vi "数据表-写入或修改记录.vi"(6 "元素名[]-探测器信息":string[](array[string]), 7 "元素名[]-累积记录":string[](array[string]), 8 "error in (no error)":errorcluster, 9 "表名-设备表":string, 10 "写改记录数据输入":T1, 11 "数据库引用":T7) -> (0 "error out":errorcluster, 1 "输出簇":T1, 2 "累积剂量增量":dbl, 3 "connection reference out":T7)   [LabVIEW 2017]
uses:
  <vilib>/addons/database/Connection.llb/Conn ObjectReference.ctl
  <vilib>/addons/database/NI_Database_API.lvlib
panel:
  out "Result 2":string caption="设备表sql-update"
  out "Result":string caption="数据表sql-update"
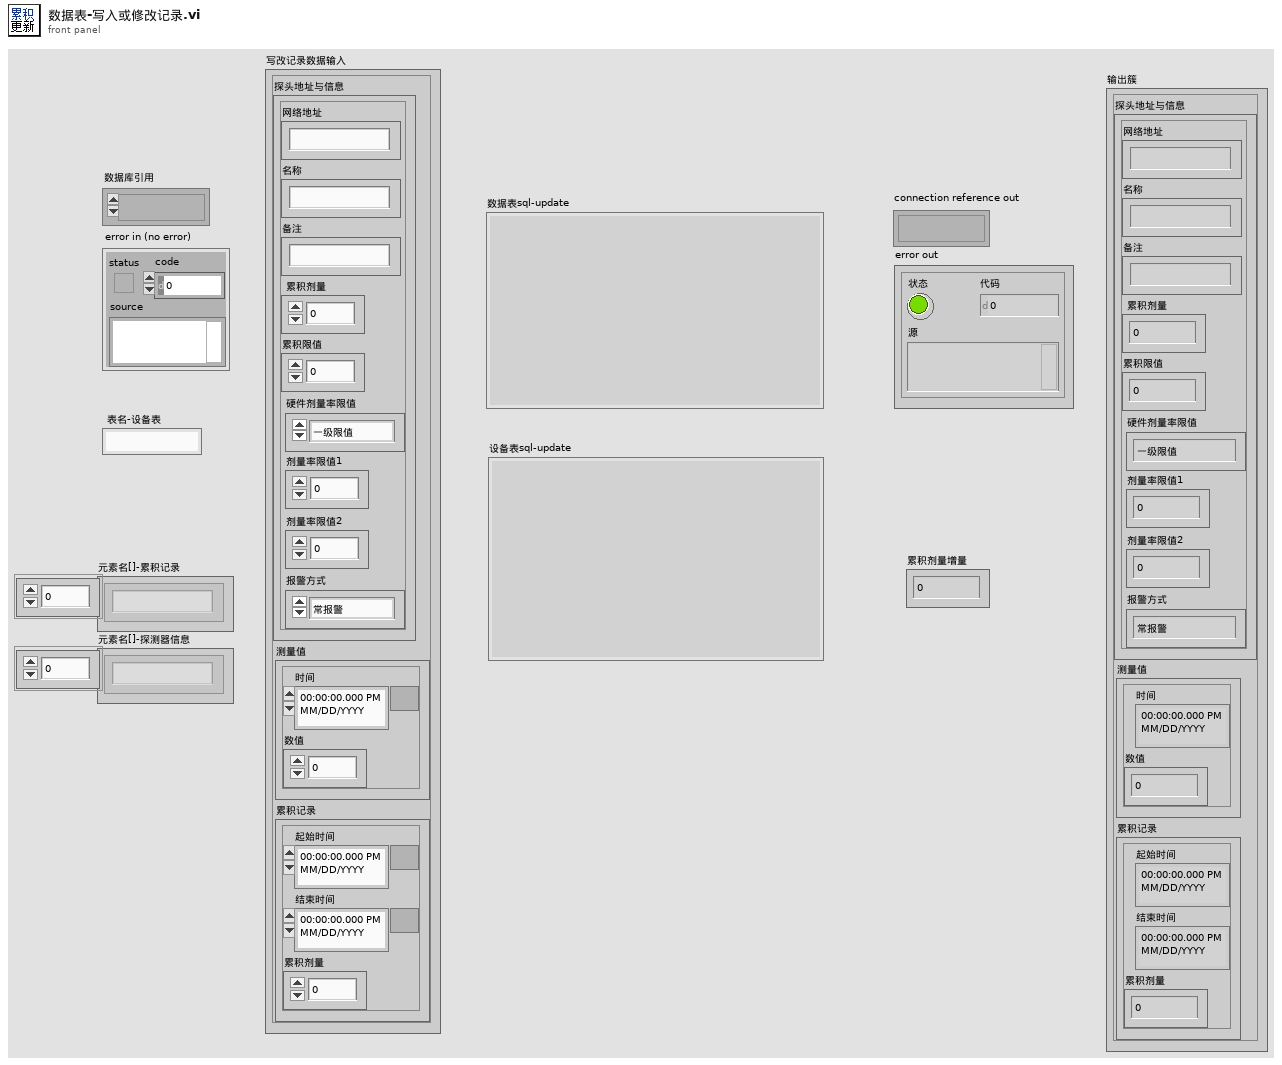
[diagram p1: front panel]
types:
  T1 = typedef "写改累积记录输入.ctl" = cluster{"探头地址与信息":T2, "测量值":T5, "累积记录":T6}
  T2 = typedef "探测器信息.ctl" = cluster{"网络地址":string, "名称":string, "备注":string, "累积剂量":dbl, "累积限值":dbl, "硬件剂量率限值":T3, "剂量率限值1":dbl, "剂量率限值2":dbl, "报警方式":T4}
  T3 = typedef "探头剂量率限值选择.ctl" = enum16{"一级限值", "二级限值"}
  T4 = typedef "报警方式选择.ctl" = enum16{"常报警", "自动静音", "手动静音"}
  T5 = typedef "测量值.ctl" = cluster{"时间":timestamp, "数值":dbl}
  T6 = typedef "单条累积记录.ctl" = cluster{"起始时间":timestamp, "结束时间":timestamp, "累积剂量":dbl}
  T7 = typedef "NI_Database_API.lvlib/Conn ObjectReference.ctl" = refnum<k1>
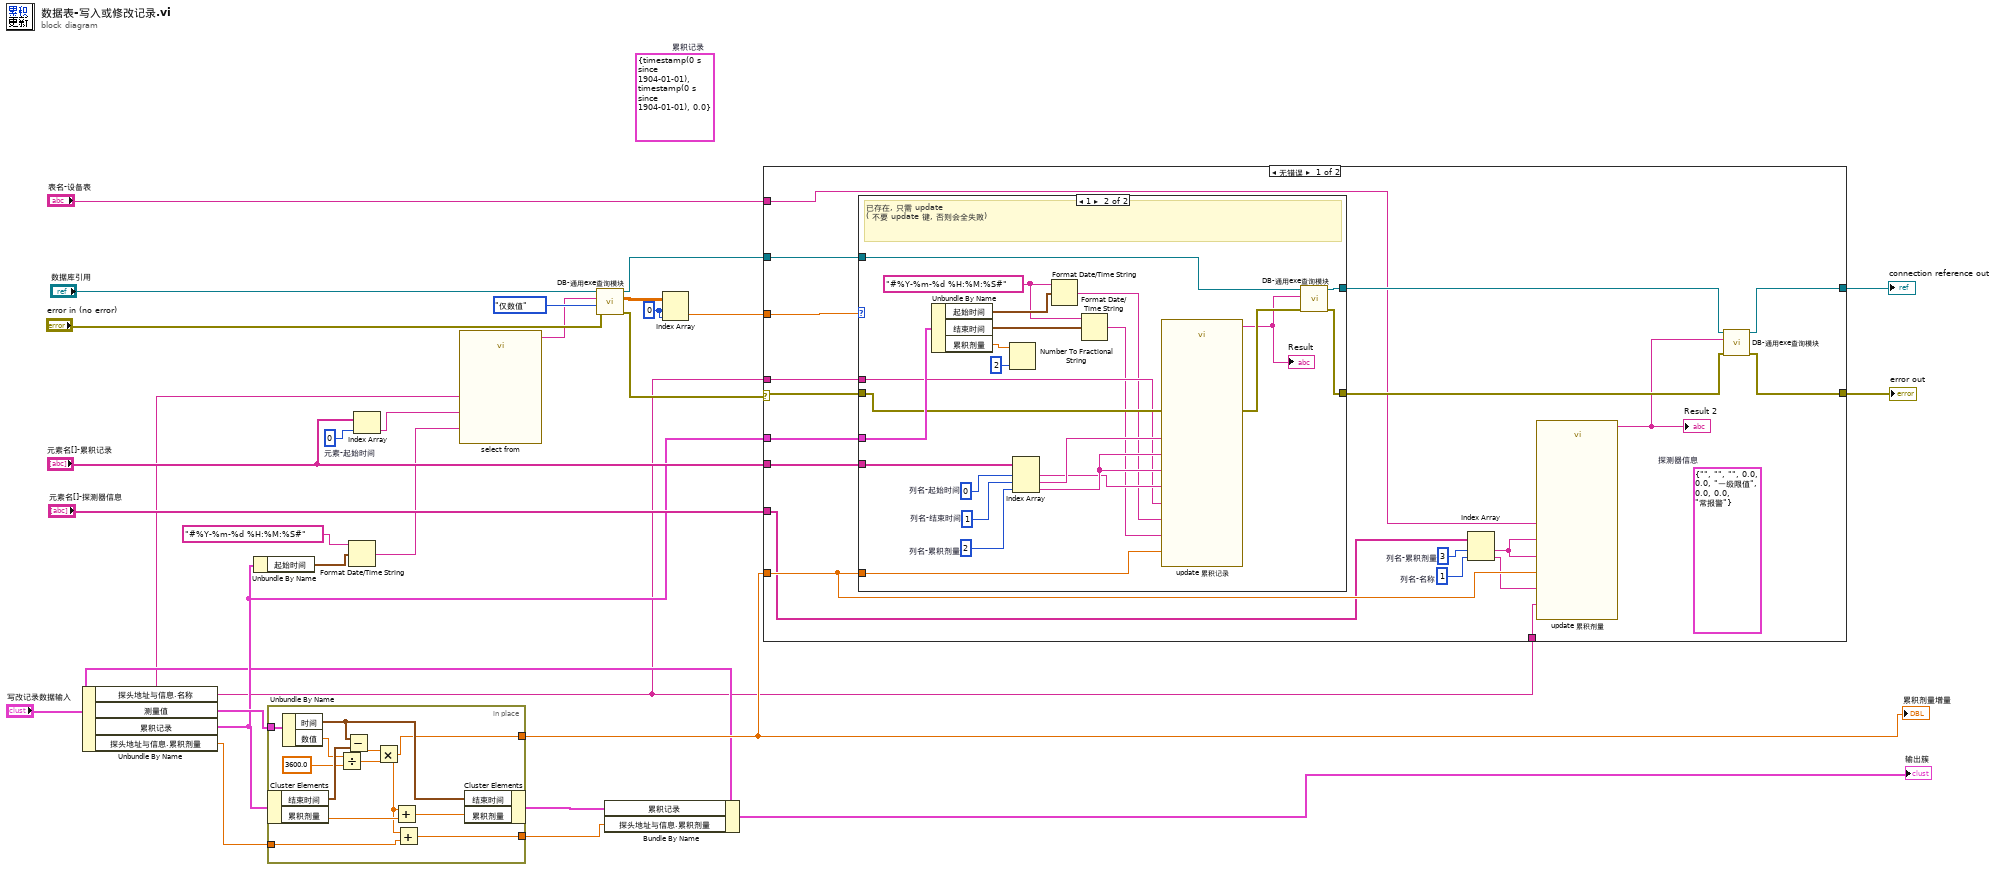
[diagram p0: block diagram]
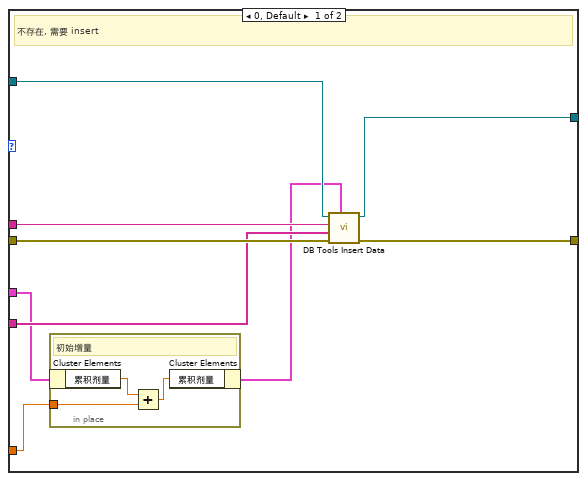
[diagram p2: hidden frame]
diagram:
  (unwired) T6 {"起始时间"=timestamp(0 s since 1904-01-01), "结束时间"=timestamp(0 s since 1904-01-01), "累积剂量"=0.0}  # 累积记录
  w22 = 0 ("索引 (行)")
  w27 = 0  # 元素-起始时间
  n1 = Unbundle By Name("写改记录数据输入") -> ("探头地址与信息.名称"=w1:string, "测量值"=w14:T5, "累积记录"=w11:T6, "探头地址与信息.累积剂量"=w3:dbl)
  n2 = Unbundle By Name(w11) -> ("起始时间"=w26:timestamp)
  n3 = in-place {
    in-place-border: w14 -> [w40]
    in-place-border: [w30] -> w7
    in-place-border: w3 -> [w31]
    in-place-border: [w29] -> w2
    n4 = in-place-cluster #1(w11) -> ("结束时间"=w38:timestamp, "累积剂量"=w39:dbl)
    n5 = Unbundle By Name(w40) -> ("时间"=w34:timestamp, "数值"=w36:dbl)
    n6 = Divide(x=w36, y=3600.0) -> (x/y=w33:dbl)
    n7 = Subtract(x=w34, y=w38) -> (x-y=w37:dbl)
    n8 = Multiply(x=w37, y=w33) -> (x*y=w30:dbl)
    n9 = Add(x=w30, y=w39) -> (x+y=w35:dbl)
    n10 = Add(x=w30, y=w31) -> (x+y=w29:dbl)
    n11 = in-place-cluster #1("结束时间"=w34, "累积剂量"=w35) -> (w5:T6)
  }
  "累积剂量增量" <- w7
  n12 = Format Date/Time String(time format string (%c)="#%Y-%m-%d %H:%M:%S#" ("时间格式字符串(%c)"), seconds (now)=w26) -> (date/time string=w9:string)  [unwired: 1 in]
  n13 = Index Array(array="元素名[]-累积记录", index=w27) -> (element=w10:string)
  n14 = call "select from"("表名"=w1, "列名-起始时间"=w9, "时间字符串"=w10) -> ("Result"=w8:string)  [unwired: 11 in, 1 out]
  n15 = call "DB-通用exe查询模块.vi"("error in (no error)"="error in (no error)", "解析模式"=enum16{"仅数值", "仅字符串", "数值与字符串"}."仅数值", "SQL query"=w8, "数据库连接引用"="数据库引用") -> ("error out"=w19:errorcluster, "数值数据"=w23:dbl[][], "数据库连接引用out"=w18:T7)  [unwired: 3 in, 2 out]
  n16 = Bundle By Name(cluster="写改记录数据输入", "累积记录"=w5, "探头地址与信息.累积剂量"=w2) -> (→"输出簇":T1)
  n17 = Index Array(array=w23, index (row)=w22, index (col)=w22) -> (element=w21:dbl)
  n18 = case shown="无错误" w19 {
    selector: w19 -> [w57 w95]
    tunnel: w21 -> [w59 _]
    tunnel: w18 -> [w58 w94]
    tunnel: [w52 w94] -> w15
    tunnel: [w50 w95] -> w17
    tunnel: w11 -> [w56 _]
    tunnel: "元素名[]-累积记录" -> [w55 _]
    tunnel: w1 -> [w54 _]
    tunnel: "元素名[]-探测器信息" -> [w47 _]
    tunnel: w7 -> [w49 _]
    tunnel: "表名-设备表" -> [w48 _]
    tunnel: w1 -> [w41 _]
    frame No Error {
      w43 = 1  # 列名-名称
      (unwired) T2 {"网络地址"="", "名称"="", "备注"="", "累积剂量"=0.0, "累积限值"=0.0, "硬件剂量率限值"=enum."一级限值", "剂量率限值1"=0.0, "剂量率限值2"=0.0, "报警方式"=enum."常报警"}  # 探测器信息
      w46 = 3  # 列名-累积剂量
      n19 = case shown="1" w59 {
        tunnel: w58 -> [w68 w92]
        tunnel: [w67 w91] -> w53
        tunnel: w57 -> [w66 w90]
        tunnel: [w65 w89] -> w51
        tunnel: w56 -> [w62 w93]
        tunnel: w55 -> [w64 w88]
        tunnel: w54 -> [w63 w80]
        tunnel: w49 -> [w61 w72]
        frame 0, Default {
          # "不存在, 需要 insert"
          n20 = in-place {
            in-place-border: w61 -> [w70]
            # "初始增量"
            n21 = in-place-cluster #2(w62) -> ("累积剂量"=w71:dbl)
            n22 = Add(x=w71, y=w70) -> (x+y=w69:dbl)
            n23 = in-place-cluster #2("累积剂量"=w69) -> (w60:T6)
          }
          n24 = call <vilib>:"DB Tools Insert Data.vi"("data"=w60, "error in (no error)"=w66, "columns"=w64, "table"=w63, "connection reference"=w68) -> ("error out"=w65:errorcluster, "connection reference out"=w67:T7)  [unwired: 5 in]
        }
        frame 1 {
          w78 = "#%Y-%m-%d %H:%M:%S#" ("时间格式字符串(%c)")
          w82 = 0  # 列名-起始时间
          w85 = 2  # 列名-累积剂量
          w86 = 1  # 列名-结束时间
          # "已存在, 只需 update\n( 不要 update 键, 否则会全失败)"
          n25 = Unbundle By Name(w93) -> ("起始时间"=w79:timestamp, "结束时间"=w77:timestamp, "累积剂量"=w76:dbl)
          n26 = Number To Fractional String(number=w76, precision (6)=i16 2 ("精度(6)")) -> ()  [unwired: 2 in, 1 out]
          n27 = Index Array(array=w88, index #1=w82, index #2=w86, index #3=w85) -> (element #1=w81:string, element #2=w84:string, element #3=w83:string)
          n28 = Format Date/Time String(time format string (%c)=w78, seconds (now)=w79) -> (date/time string=w74:string)  [unwired: 1 in]
          n29 = Format Date/Time String(time format string (%c)=w78, seconds (now)=w77) -> (date/time string=w73:string)  [unwired: 1 in]
          n30 = call "update 累积记录"("列名-累积剂量"=w83, "累积剂量增量"=w72, "起始时间"=w74, "表名-数据表"=w80, "列名-结束时间"=w84, "结束时间"=w73, "列名-累积剂量1"=w83, "列名-起始时间"=w81) -> ("Result"=w87:string)  [unwired: 6 in, 1 out]
          "Result" <- w87
          n31 = call "DB-通用exe查询模块.vi"("error in (no error)"=w90, "SQL query"=w87, "数据库连接引用"=w92) -> ("error out"=w89:errorcluster, "数据库连接引用out"=w91:T7)  [unwired: 4 in, 3 out]
        }
      }
      n32 = Index Array(array=w47, index #1=w46, index #2=w43) -> (element #1=w45:string, element #2=w42:string)
      n33 = call "update 累积剂量"("累积剂量增量"=w49, "名称"=w41, "表名-设备表"=w48, "列名-累积剂量"=w45, "列名-累积剂量1"=w45, "列名-名称"=w42) -> ("Result"=w44:string)  [unwired: 8 in, 1 out]
      "Result 2" <- w44
      n34 = call "DB-通用exe查询模块.vi"("error in (no error)"=w51, "SQL query"=w44, "数据库连接引用"=w53) -> ("error out"=w50:errorcluster, "数据库连接引用out"=w52:T7)  [unwired: 4 in, 3 out]
    }
    frame Error {
    }
  }
  "connection reference out" <- w15
  "error out" <- w17
